vi "Get trap pos.vi"(2 "Switch X/Y":bool, 3 "ROI":T1) -> (0 "Trap positions Y (IMAQ coordinates)":i32[](array[numeric]), 1 "Trap positions X (IMAQ coordinates)":i32[](array[numeric]))   [LabVIEW 2012]
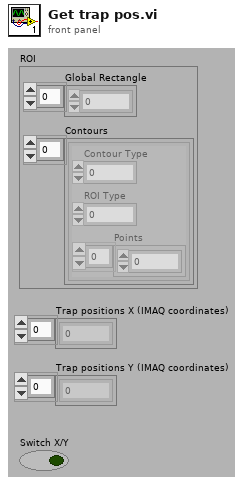
[diagram p1: front panel]
types:
  T1 = cluster{"Global Rectangle":i32[], "Contours":cluster{"Contour Type":u32, "ROI Type":u32, "Points":i32[]}[]}
  T2 = cluster{"Contour Type":u32, "ROI Type":u32, "Points":i32[]}[]
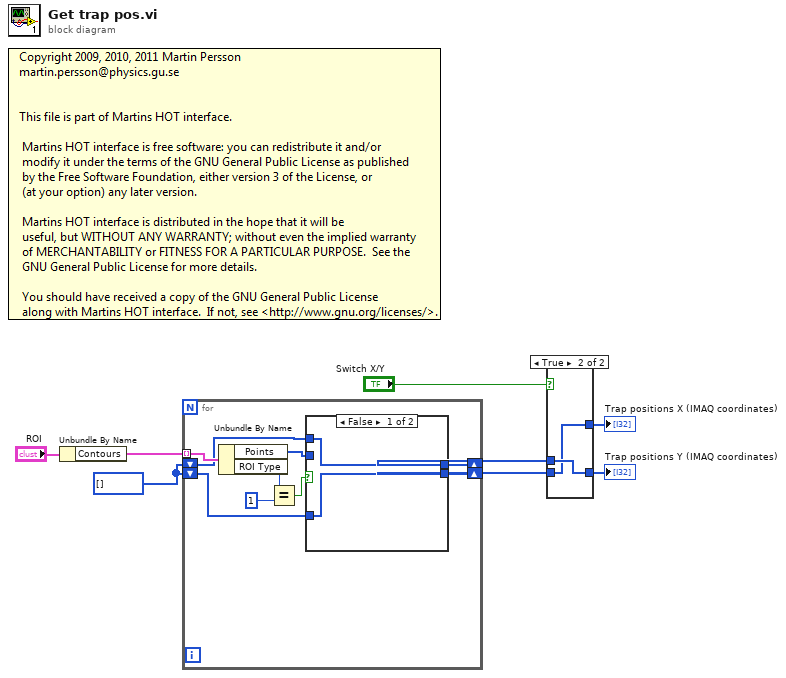
[diagram p0: block diagram]
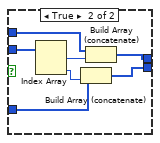
[diagram p3: hidden frame]
diagram:
  w1 = i32[] []
  n1 = Unbundle By Name("ROI") -> ("Contours"=w8:T2)
  n2 = for {
    tunnel: w8 -> [w17] mode=indexing
    shift-right: [w13] -> w6
    shift-left: w1 -> [w12]
    shift-right: [w11] -> w4
    shift-left: w1 -> [w10]
    n3 = Unbundle By Name(w17) -> ("Points"=w16:i32[], "ROI Type"=w15:u32)
    n4 = Equal?(x=w15, y=u32 1) -> (x = y?=w9:bool)
    n5 = case shown="False" w9 {
      tunnel: w16 -> [_ w26]
      tunnel: [w19 w24] -> w13
      tunnel: w12 -> [w19 w23]
      tunnel: [w18 w21] -> w11
      tunnel: w10 -> [w18 w20]
      frame False {
      }
      frame True {
        n6 = Index Array(array=w26) -> (element #1=w25:i32, element #2=w22:i32)  [unwired: 2 in]
        n7 = Build Array (concatenate)(w20, w22) -> (w21:i32[])
        n8 = Build Array (concatenate)(w23, w25) -> (w24:i32[])
      }
    }
  }
  n9 = case shown="True" "Switch X/Y" {
    tunnel: w6 -> [w28 w30]
    tunnel: [w27 w30] -> w5
    tunnel: w4 -> [w27 w29]
    tunnel: [w28 w29] -> w3
    frame False {
    }
    frame True {
    }
  }
  "Trap positions Y (IMAQ coordinates)" <- w5
  "Trap positions X (IMAQ coordinates)" <- w3
